vi "Write to Hardware.vi"(7 "Valid Triggers":bool, 8 "error in":errorcluster, 9 "Trigger Values":dbl[](array[numeric]), 10 "Values":dbl[](array[numeric]), 11 "Tx Execution Unit Implementation in":refnum<class "Tx Execution Unit.lvclass">) -> (0 "error out":errorcluster, 1 "Trigger Values out":dbl[](array[numeric]), 2 "Values out":dbl[](array[numeric]), 3 "Tx Execution Unit Implementation out":refnum<class "Tx Execution Unit.lvclass">)   [LabVIEW 2023, in "Ballard MIL-STD-1553 Engine Support.lvlib" / "Implementation.lvlib" / "Tx Execution Unit.lvclass"]
uses:
  Tx Execution Unit.lvclass
  Tx Execution Unit.lvclass/Tx Execution Unit.ctl
  Encode Parameters to Words.vi/57287a39-98a1-4235-a14c-2bf7a66eb33b.vi
  Encode Parameters to Words.vi/3ea03746-6f70-437b-b143-209d604836ee.vi
  Encode Parameters to Words.vi/57287a39-98a1-4235-a14c-2bf7a66eb33b.vi/136dcdcb-2dd3-4a4d-a796-a8f7a3f8e1ac.vi
  Encode Parameters to Words.vi/57287a39-98a1-4235-a14c-2bf7a66eb33b.vi/a54b505c-1216-4ef4-8378-3ceda9d188df.vi
  Encode Parameters to Words.vi/3ea03746-6f70-437b-b143-209d604836ee.vi/9377bb8f-44b5-4a8f-87f1-966fd5a9edcc.vi
  Encode Parameters to Words.vi/3ea03746-6f70-437b-b143-209d604836ee.vi/e95d9d1f-307c-44d6-9f26-c3f519a4990d.vi
  Encode Parameters to Words.vi/3ea03746-6f70-437b-b143-209d604836ee.vi/0c23f515-4369-4514-bc3d-4444e6b437b2.vi
  <vilib>/NI/NI VeriStand Encoding and Decoding/Get Bits Per Digit from Base.vi
  Scripting/Constants.vi
  <instrlib>/BTI1553Lib/BTI1553LV.lvlib
  Scripting/Ballard MIL-STD-1553 Scripting.lvlib
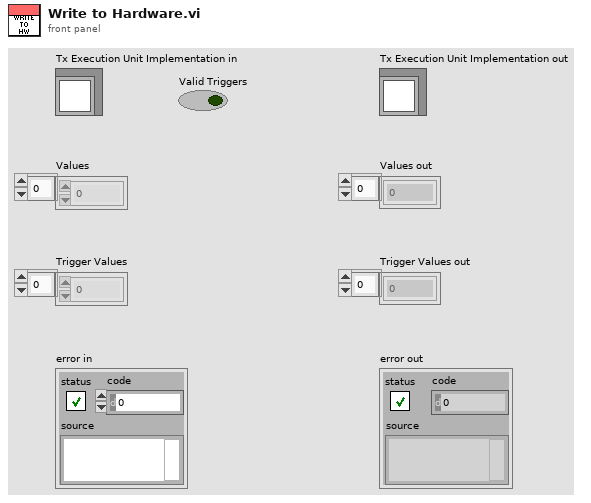
[diagram p1: front panel]
types:
  T1 = typedef "Tx Write Info.ctl" = cluster{"transfer handle":u64, "value index":i32}
  T2 = typedef "Message Definition.ctl" = cluster{"name":string, "message type":T3, "endpoint Tx":T4, "endpoint Rx":T4, "create timestamp channel":bool, "mode code":u16, "number of words":u16, "parameters":cluster{"name":string, "default value":dbl, "unit":string, "parameter definition":T6}[]}
  T3 = typedef "Message Type.ctl" = string
  T4 = typedef "Terminal Endpoint.ctl" = cluster{"terminal address":T5, "subaddress":T5}
  T5 = typedef "Address.ctl" = u16
  T6 = typedef "Parameter Definition.ctl" = cluster{"start index":i32, "size (bits)":i32, "encoding":enum16{"BNR", "BCD", "Discrete"}, "signed":bool, "multiplier":dbl, "offset":dbl}
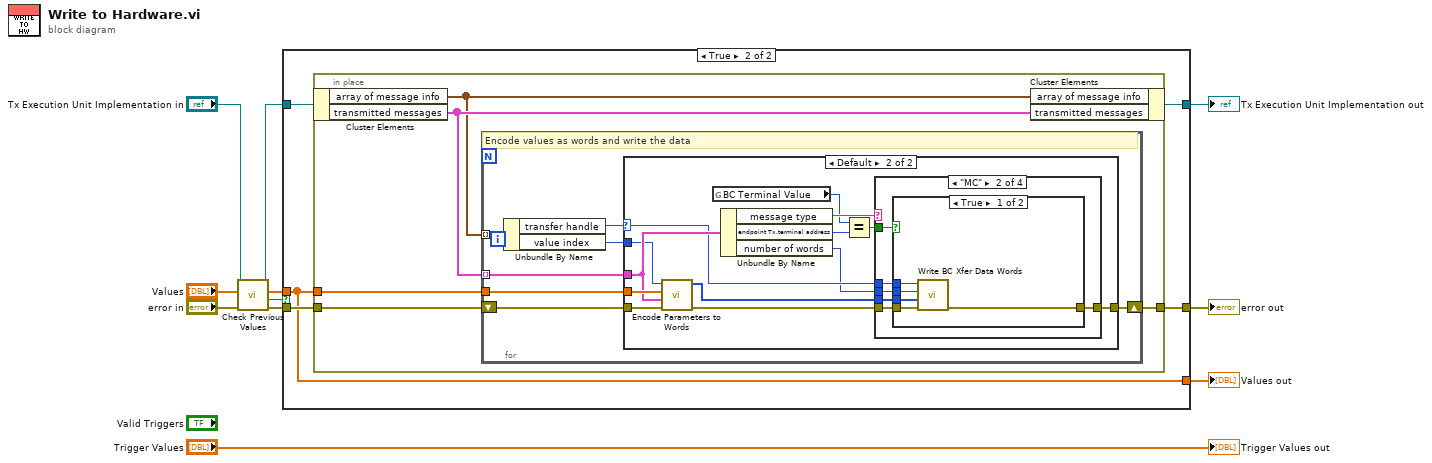
[diagram p0: block diagram]
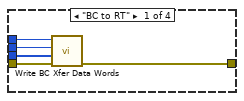
[diagram p4: hidden frame]
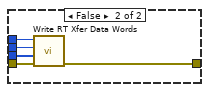
[diagram p5: hidden frame]
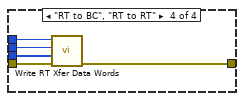
[diagram p7: hidden frame]
diagram:
  n1 = call-dynamic "Check Previous Values.vi"("error in"="error in", "values"="Values", "Tx Execution Unit Implementation in"="Tx Execution Unit Implementation in") -> ("error out"=w1:errorcluster, "values modified?"=w7:bool, "values out"=w8:dbl[], "Tx Execution Unit Implementation out"=w4:refnum<class "Tx Execution Unit.lvclass">)  [unwired: 5 in]
  n2 = case shown="True" w7 {
    tunnel: [w13 w19] -> w10
    tunnel: w4 -> [w14 w17]
    tunnel: w1 -> [w13 w18]
    tunnel: [w14 w16] -> w3
    tunnel: w8 -> [w12 w15]
    tunnel: [w12 w15] -> w9
    frame False {
    }
    frame True {
      n3 = in-place {
        in-place-border: [w24] -> w19
        in-place-border: w18 -> [w23]
        in-place-border: w15 -> [w22]
        n4 = in-place-cluster #1(w17) -> ("array of message info"=w20:T1[], "transmitted messages"=w21:T2[])
        n5 = for {
          shift-right: [w31] -> w24
          shift-left: w23 -> [w30]
          tunnel: w21 -> [w28] mode=indexing
          tunnel: w22 -> [w29]
          tunnel: w20 -> [w25] mode=indexing
          # "Encode values as words and write the data"
          n6 = Unbundle By Name(w25) -> ("transfer handle"=w27:u64, "value index"=w26:i32)
          n7 = case shown="Default" w27 {
            selector: w27 -> [_ w43]
            tunnel: w29 -> [_ w45]
            tunnel: w28 -> [_ w44]
            tunnel: w26 -> [_ w42]
            tunnel: [w32 w39] -> w31
            tunnel: w30 -> [w32 w38]
            frame 0, -1 {
            }
            frame Default {
              n8 = call "Encode Parameters to Words.vi"("error in"=w38, "message"=w44, "Values"=w45, "value index"=w42) -> ("error out"=w37:errorcluster, "data words"=w40:u16[])  [unwired: 6 in]
              n9 = global read "Constants.vi" "BC Terminal Value"() -> (w35:u16)
              n10 = Unbundle By Name(w44) -> ("message type"=w36:T3, "endpoint Tx.terminal address"=w34:T5, "number of words"=w41:u16)
              n11 = Equal?(x=w35, y=w34) -> (x = y?=w33:bool)
              n12 = case shown="\"MC\"" w36 {
                tunnel: [w46 w52 w67 w72] -> w39
                tunnel: w41 -> [w48 w54 _ w71]
                tunnel: w43 -> [w47 w53 _ w70]
                tunnel: w40 -> [w49 w55 _ w69]
                tunnel: w37 -> [w50 w56 w67 w68]
                tunnel: w33 -> [_ w51 _ _]
                frame "BC to RT" {
                  n13 = call <instrlib>:"Write BC Xfer Data Words.vi"("error in (no error)"=w50, "data words"=w49, "data word count in"=w48, "bc transfer handle in"=w47) -> ("error out"=w46:errorcluster)  [unwired: 5 in, 2 out]
                }
                frame "MC" {
                  n14 = case shown="True" w51 {
                    tunnel: w56 -> [w61 w66]
                    tunnel: w55 -> [w60 w62]
                    tunnel: w54 -> [w59 w63]
                    tunnel: w53 -> [w58 w64]
                    tunnel: [w57 w65] -> w52
                    frame True {
                      n15 = call <instrlib>:"Write BC Xfer Data Words.vi"("error in (no error)"=w61, "data words"=w60, "data word count in"=w59, "bc transfer handle in"=w58) -> ("error out"=w57:errorcluster)  [unwired: 5 in, 2 out]
                    }
                    frame False {
                      n16 = call <instrlib>:"Write RT Xfer Data Words.vi"("error in (no error)"=w66, "data words"=w62, "data word count in"=w63, "rt transfer handle in"=w64) -> ("error out"=w65:errorcluster)  [unwired: 5 in, 2 out]
                    }
                  }
                }
                frame Default {
                }
                frame "RT to BC", "RT to RT" {
                  n17 = call <instrlib>:"Write RT Xfer Data Words.vi"("error in (no error)"=w68, "data words"=w69, "data word count in"=w71, "rt transfer handle in"=w70) -> ("error out"=w72:errorcluster)  [unwired: 5 in, 2 out]
                }
              }
            }
          }
        }
        n18 = in-place-cluster #1("array of message info"=w20, "transmitted messages"=w21) -> (w16:refnum<class "Tx Execution Unit.lvclass">)
      }
    }
  }
  "error out" <- w10
  "Tx Execution Unit Implementation out" <- w3
  "Values out" <- w9
  "Trigger Values out" <- "Trigger Values"
